vi "SP Append Adapter Waveforms.vi"(7 "Attribute Name (NI_ChannelName)":string="NI_ChannelName", 8 "error in (no error)":errorcluster, 10 "Adapters":T1[](array[typedef]), 11 "Waveforms in":waveform(dbl)[](array[waveform])) -> (0 "error out":errorcluster, 3 "Waveforms out":waveform(dbl)[](array[waveform]))   [LabVIEW 2011]
uses:
  TypeDefs/SP Adapter.ctl
  TypeDefs/SP Data.ctl
  TypeDefs/SP Channel Type.ctl
  TypeDefs/SP Format.ctl
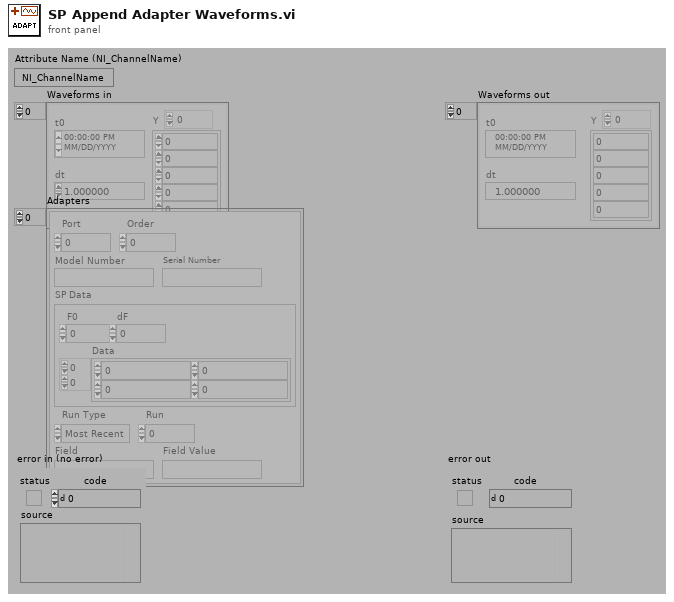
[diagram p1: front panel]
types:
  T1 = typedef "SP Adapter.ctl" = cluster{"Port":i8, "Order":i8, "Model Number":string, "Serial Number":string, "SP Data":T2, "Run Type":enum16{"Most Recent", "Run #", "Match Field"}, "Run":i32, "Field":string, "Field Value":string}
  T2 = typedef "SP Data.ctl" = cluster{"F0":dbl, "dF":dbl, "Data":cdb[][]}
  T3 = typedef "SP Format.ctl" = enum16{"Log Mag", "Lin Mag", "SWR", "Phase", "Expanded Phase", "Delay", "Insertion Loss", "Isolation", "Return Loss"}
  T4 = typedef "SP Channel Type.ctl" = enum16{"Frequency", "Data", "Limit", "Adapter", "Memory", "Value", "Value Limit"}
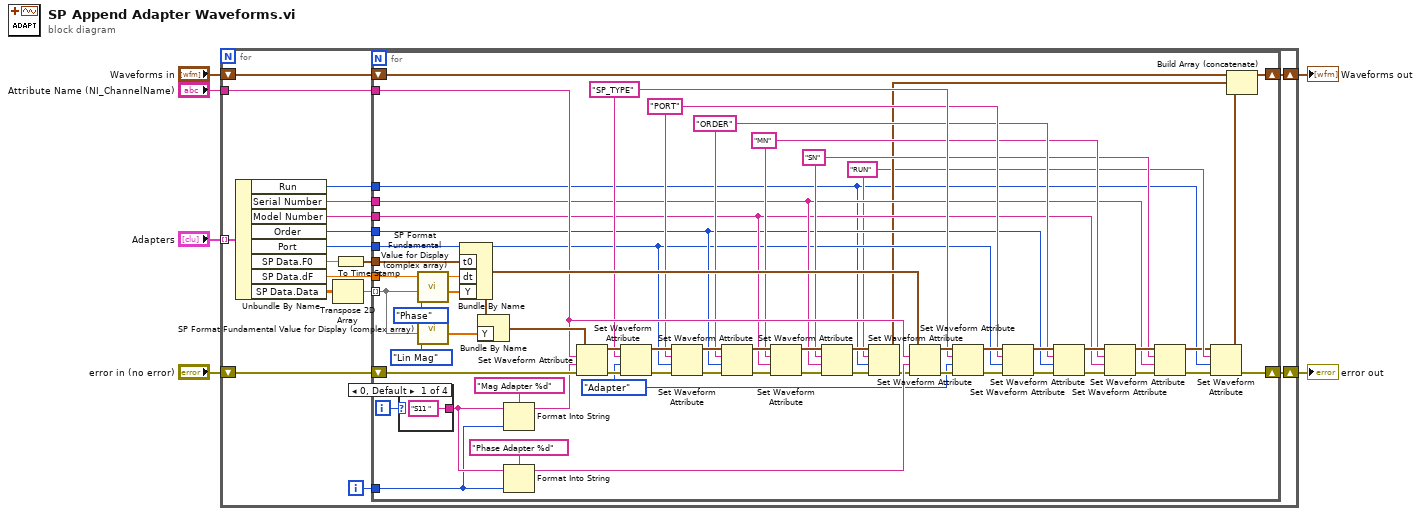
[diagram p0: block diagram]
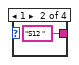
[diagram p2: hidden frame]
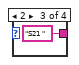
[diagram p3: hidden frame]
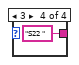
[diagram p4: hidden frame]
diagram:
  n1 = for {
    tunnel: "Adapters" -> [w21] mode=indexing
    shift-right: [w22] -> w4
    shift-left: "error in (no error)" -> [w23]
    tunnel: "Attribute Name (NI_ChannelName)" -> [w14]
    shift-right: [w12] -> w1
    shift-left: "Waveforms in" -> [w13]
    i -> [w15]
    n2 = Unbundle By Name(w21) -> ("Run"=w7:i32, "Serial Number"=w8:string, "Model Number"=w9:string, "Order"=w10:i8, "Port"=w11:i8, "SP Data.F0"=w20:dbl, "SP Data.dF"=w18:dbl, "SP Data.Data"=w17:cdb[][])
    n3 = Transpose 2D Array(2D array=w17) -> (transposed array=w16:cdb[][])
    n4 = To Time Stamp(1:w20) -> (0:w19:timestamp)
    n5 = for {
      tunnel: w19 -> [w82]
      tunnel: w18 -> [w81]
      shift-right: [w26] -> w22
      shift-left: w23 -> [w83]
      tunnel: w16 -> [w78] mode=indexing
      tunnel: w15 -> [w71]
      tunnel: w14 -> [w66]
      shift-right: [w65] -> w12
      shift-left: w13 -> [w64]
      tunnel: w11 -> [w34]
      tunnel: w10 -> [w35]
      tunnel: w9 -> [w36]
      tunnel: w8 -> [w37]
      tunnel: w7 -> [w24]
      i -> [w72]
      w29 = "RUN" ("format string")
      w38 = "SN" ("format string")
      w39 = "MN" ("format string")
      w40 = "ORDER" ("format string")
      w41 = "PORT" ("format string")
      w58 = "SP_TYPE" ("format string")
      w59 = SP_Channel_Type."Adapter" ("Channel Type")
      n6 = case shown="0, Default" w72 {
        tunnel: ["S11 " ("format string") "S12 " ("format string") "S21 " ("format string") "S22 " ("format string")] -> w75
        frame 0, Default {
        }
        frame 1 {
        }
        frame 2 {
        }
        frame 3 {
        }
      }
      n7 = call "SP Format Fundamental Value for Display (complex array).vi"("Sxx Measured Format"=SP_Format."Phase" ("Sxx Measure Format"), "Fundamental Values"=w78) -> ("Formatted Values"=w77:dbl[])  [unwired: 1 in, 8 out]
      n8 = call "SP Format Fundamental Value for Display (complex array).vi"("Sxx Measured Format"=SP_Format."Lin Mag" ("Sxx Measure Format"), "Fundamental Values"=w78) -> ("Formatted Values"=w76:dbl[])  [unwired: 1 in, 8 out]
      n9 = Bundle By Name("t0"=w82, "dt"=w81, "Y"=w77) -> (w67:waveform(dbl))  [unwired: 1 out]
      n10 = Bundle By Name(cluster=w67, "Y"=w76) -> (w69:waveform(dbl))
      n11 = Format Into String(format string="Mag Adapter %d", initial string=w75, w71) -> (resulting string=w70:string)  [unwired: 1 in, 1 out]
      n12 = Format Into String(format string="Phase Adapter %d", initial string=w75, w71) -> (resulting string=w68:string)  [unwired: 1 in, 1 out]
      n13 = Set Waveform Attribute(4:w83, 5:w70, 6:w66, 7:w69) -> (0:w63:errorcluster, 3:w62:waveform(dbl))  [unwired: 1 out]
      n14 = Set Waveform Attribute(4:w63, 5:w59, 6:w58, 7:w62) -> (0:w57:errorcluster, 3:w42:waveform(dbl))  [unwired: 1 out]
      n15 = Set Waveform Attribute(4:w57, 5:w34, 6:w41, 7:w42) -> (0:w56:errorcluster, 3:w43:waveform(dbl))  [unwired: 1 out]
      n16 = Set Waveform Attribute(4:w56, 5:w35, 6:w40, 7:w43) -> (0:w55:errorcluster, 3:w44:waveform(dbl))  [unwired: 1 out]
      n17 = Set Waveform Attribute(4:w55, 5:w36, 6:w39, 7:w44) -> (0:w54:errorcluster, 3:w45:waveform(dbl))  [unwired: 1 out]
      n18 = Set Waveform Attribute(4:w54, 5:w37, 6:w38, 7:w45) -> (0:w30:errorcluster, 3:w33:waveform(dbl))  [unwired: 1 out]
      n19 = Set Waveform Attribute(4:w30, 5:w24, 6:w29, 7:w33) -> (0:w31:errorcluster, 3:w32:waveform(dbl))  [unwired: 1 out]
      n20 = Set Waveform Attribute(4:w31, 5:w68, 6:w66, 7:w67) -> (0:w61:errorcluster, 3:w60:waveform(dbl))  [unwired: 1 out]
      n21 = Set Waveform Attribute(4:w61, 5:w59, 6:w58, 7:w60) -> (0:w53:errorcluster, 3:w46:waveform(dbl))  [unwired: 1 out]
      n22 = Set Waveform Attribute(4:w53, 5:w34, 6:w41, 7:w46) -> (0:w52:errorcluster, 3:w47:waveform(dbl))  [unwired: 1 out]
      n23 = Set Waveform Attribute(4:w52, 5:w35, 6:w40, 7:w47) -> (0:w51:errorcluster, 3:w48:waveform(dbl))  [unwired: 1 out]
      n24 = Set Waveform Attribute(4:w51, 5:w36, 6:w39, 7:w48) -> (0:w50:errorcluster, 3:w49:waveform(dbl))  [unwired: 1 out]
      n25 = Set Waveform Attribute(4:w50, 5:w37, 6:w38, 7:w49) -> (0:w28:errorcluster, 3:w27:waveform(dbl))  [unwired: 1 out]
      n26 = Set Waveform Attribute(4:w28, 5:w24, 6:w29, 7:w27) -> (0:w26:errorcluster, 3:w25:waveform(dbl))  [unwired: 1 out]
      n27 = Build Array (concatenate)(w64, w32, w25) -> (w65:waveform(dbl)[])
    }
  }
  "Waveforms out" <- w1
  "error out" <- w4
